vi "rtd.vi"() -> ()   [LabVIEW 2024]
panel:
  in  "?":bool
  out "Waveform Chart":dbl[][](graph)
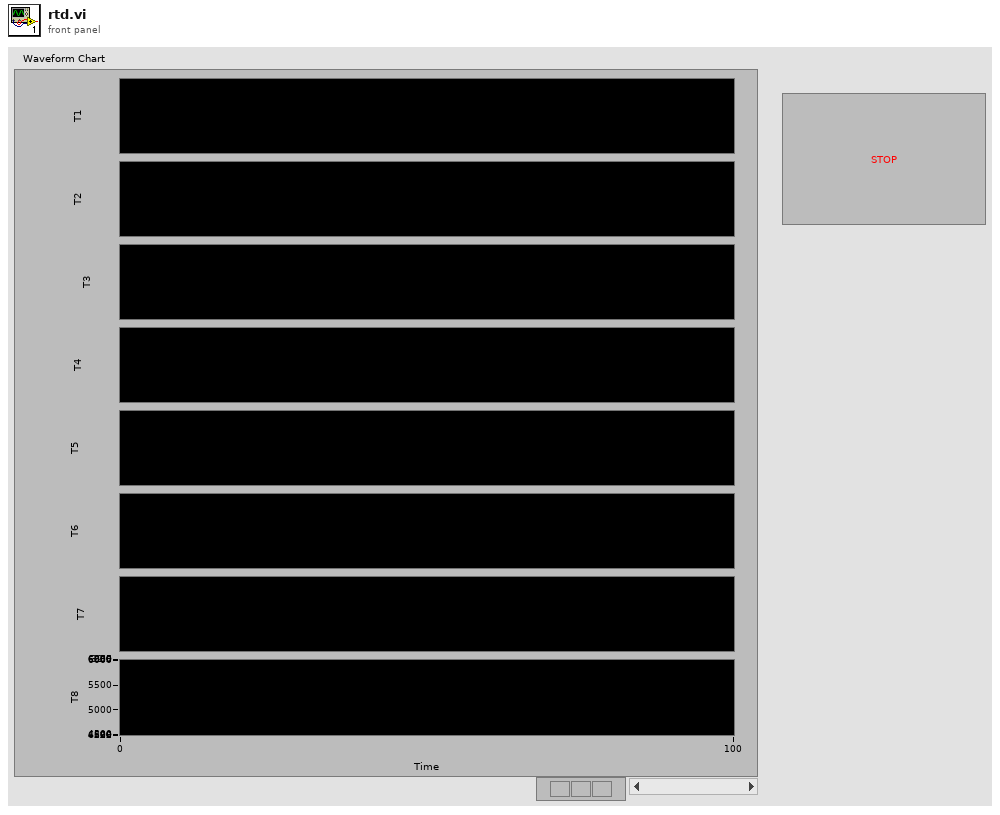
[diagram p1: front panel]
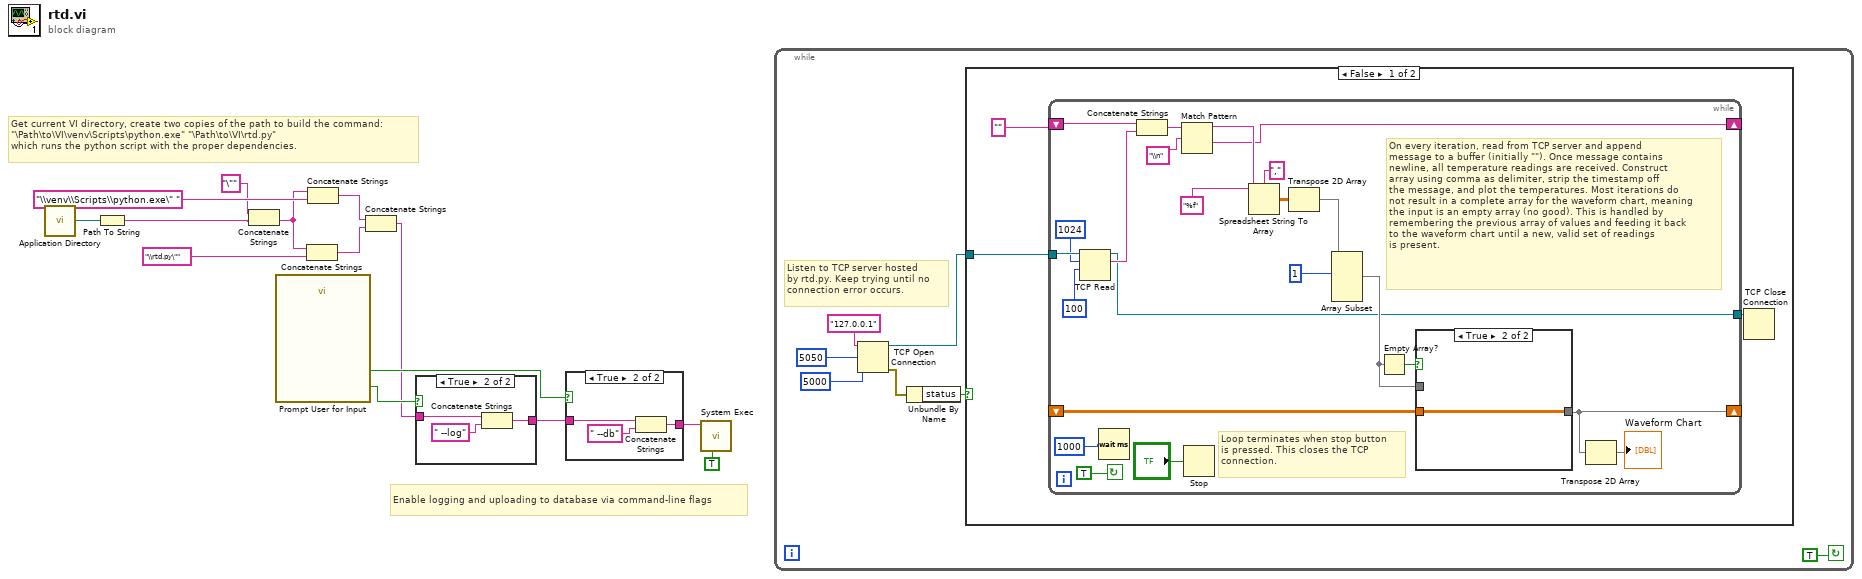
[diagram p0: block diagram]
diagram:
  # "Enable logging and uploading to database via command-line flags"
  # "Get current VI directory, create two copies of the path to build the command:\n\"\\Path\\to\\VI\\venv\\Scripts\\python.exe\" \"\\Path\\to\\VI\\rtd.py\"\nwhich runs the python script with the proper dependencies."
  n1 = call <vilib>:"Application Directory.vi"() -> ("Application Directory"=w1:path)
  n2 = Path To String(path=w1) -> (string=w2:string)
  n3 = Concatenate Strings("\"" ("string"), w2) -> (w6:string)
  n4 = call "Prompt User for Input"() -> ("Record logging information?"=w14:bool, "Record session to database?"=w13:bool)  [unwired: 16 in, 2 out]
  n5 = Concatenate Strings(w6, "\\rtd.py\"" ("string")) -> (w4:string)
  n6 = Concatenate Strings(w6, "\\venv\\Scripts\\python.exe\" " ("string")) -> (w5:string)
  n7 = Concatenate Strings(w5, w4) -> (w3:string)
  n8 = case shown="True" w14 {
    tunnel: w3 -> [w15 w18]
    tunnel: [w15 w16] -> w11
    frame False {
    }
    frame True {
      n9 = Concatenate Strings(w18, " --log") -> (w16:string)
    }
  }
  n10 = case shown="True" w13 {
    tunnel: w11 -> [w19 w21]
    tunnel: [w19 w20] -> w12
    frame False {
    }
    frame True {
      n11 = Concatenate Strings(w21, " --db") -> (w20:string)
    }
  }
  n12 = call <vilib>:"System Exec.vi"("run minimized? (F)"=TRUE, "command line"=w12) -> ()  [unwired: 6 in, 4 out]
  n13 = while {
    stop <- TRUE continue-if-true
    # "Listen to TCP server hosted\nby rtd.py. Keep trying until no\nconnection error occurs."
    n14 = TCP Open Connection(address="127.0.0.1", remote port or service name=u16 5050, timeout ms (60000)=5000) -> (connection ID=w26:refnum<k5>, error out=w25:errorcluster)  [unwired: 2 in]
    n15 = Unbundle By Name(w25) -> ("status"=w24:bool)
    n16 = case shown="False" w24 {
      tunnel: w26 -> [w31 _]
      frame False {
        n17 = while {
          tunnel: w31 -> [w55]
          shift-right: [w36] -> _
          shift-left: "" -> [w53]
          shift-right: [w40] -> _
          shift-left: _ -> [w41]
          tunnel: [w35] -> w30
          stop <- TRUE continue-if-true
          # "Loop terminates when stop button\nis pressed. This closes the TCP\nconnection."
          # "On every iteration, read from TCP server and append \nmessage to a buffer (initially \"\"). Once message contains\nnewline, all temperature readings are received. Construct \narray using comma as delimiter, strip the timestamp off\nthe message, and plot the temperatures. Most iterations do \nnot result in a complete array for the waveform chart, meaning\nthe input is an empty array (no good). This is handled by \nremembering the previous array of values and feeding it back \nto the waveform chart until a new, valid set of readings\nis present."
          n18 = TCP Read(connection ID=w55, bytes to read=1024, 9:100 ("timeout ms (25000)")) -> (connection ID out=w35:refnum<k5>, data out=w38:string)  [unwired: 2 in, 1 out]
          n19 = Wait (ms)(milliseconds to wait=u32 1000) -> ()  [unwired: 1 out]
          n20 = Concatenate Strings(w53, w38) -> (w52:string)
          n21 = Match Pattern(string=w52, regular expression="\\n") -> (before substring=w49:string, after substring=w36:string)  [unwired: 1 in, 2 out]
          n22 = Stop(stop? (T)="?") -> ()
          n23 = Spreadsheet String To Array(delimiter (Tab)=",", format string="%f", spreadsheet string=w49) -> (array=w46:dbl[][])  [unwired: 1 in]
          n24 = Transpose 2D Array(2D array=w46) -> (transposed array=w45:dbl[][])
          n25 = Array Subset(array=w45, index (row)=1 ("index")) -> (w42:dbl[][])  [unwired: 3 in]
          n26 = Empty Array?(array=w42) -> (empty?=w43:bool)
          n27 = case shown="True" w43 {
            tunnel: w42 -> [w56 _]
            tunnel: w41 -> [_ w57]
            tunnel: [w56 w57] -> w40
            frame False {
            }
            frame True {
            }
          }
          n28 = Transpose 2D Array(2D array=w40) -> (transposed array=→"Waveform Chart":dbl[][])
        }
        n29 = TCP Close Connection(connection ID=w30) -> ()  [unwired: 2 in, 2 out]
      }
      frame True {
        # "When there is a connection error, do nothing and try again"
      }
    }
  }
